vi "Perform Action.vi"(8 "error in (no error)":errorcluster, 11 "Device in":refnum<class "Device.lvclass">) -> (0 "error out":errorcluster, 3 "Device out":refnum<class "Device.lvclass">)   [LabVIEW 2020, in "Device.lvlib" / "Device.lvclass"]
uses:
  Device.lvclass
  Device.lvclass/Device.ctl
  <vilib>/ActorFramework/Message Enqueuer/Message Enqueuer.lvclass/Message Enqueuer.ctl
  <vilib>/ActorFramework/Message Enqueuer/Enqueue.vi
  Device Messages/Perform Action Msg/Perform Action Msg.lvclass
  C:/Program Files (x86)/National Instruments/LabVIEW 2020/vi.lib/ActorFramework/Message/Message.lvclass
  <vilib>/ActorFramework/Message Priority Queue/Priority Enqueue.vi
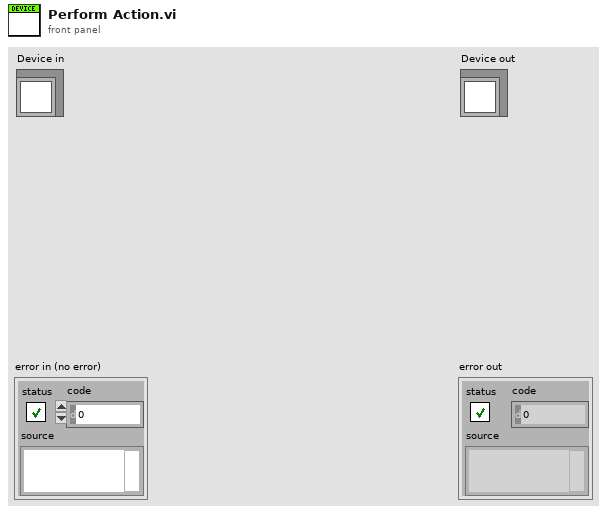
[diagram p1: front panel]
types:
  T1 = typedef "Device.lvlib/Device.lvclass/cyclical pattern.ctl" = enum16{"No Loop", "Fastest", "Timer"}
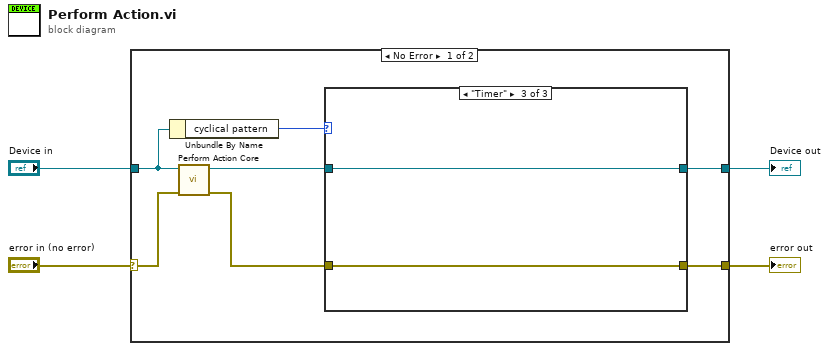
[diagram p0: block diagram]
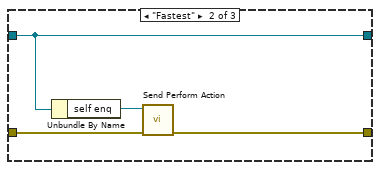
[diagram p3: hidden frame]
diagram:
  n1 = case shown="No Error" "error in (no error)" {
    selector: "error in (no error)" -> [w11 w21]
    tunnel: [w10 w21] -> w3
    tunnel: [w5 w20] -> w1
    tunnel: "Device in" -> [w8 w20]
    frame No Error {
      n2 = Unbundle By Name(w8) -> ("cyclical pattern"=w7:T1)
      n3 = call-dynamic "Perform Action Core.vi"("error in (no error)"=w11, "Device in"=w8) -> ("error out"=w9:errorcluster, "Device out"=w6:refnum<class "Device.lvclass">)  [unwired: 8 in]
      n4 = case shown="\"Timer\"" w7 {
        tunnel: [w12 w16 w18] -> w10
        tunnel: w9 -> [w12 w17 w18]
        tunnel: w6 -> [w13 w15 w19]
        tunnel: [w13 w15 w19] -> w5
        frame "No Loop", Default {
        }
        frame "Fastest" {
          n5 = Unbundle By Name(w15) -> ("self enq"=w14:refnum<class "Message Enqueuer.lvclass">)
          n6 = call "Send Perform Action.vi"("error in (no error)"=w17, "Message Enqueuer"=w14) -> ("error out"=w16:errorcluster)  [unwired: 8 in, 1 out]
        }
        frame "Timer" {
        }
      }
    }
    frame Error {
    }
  }
  "error out" <- w3
  "Device out" <- w1
